vi "Gase und Konzentrationen splitten.vi"(11 "Empfangsdaten (Eingang)":string[](array[string])) -> (1 "Konzentrationen":string[](array[string]), 2 "Gase":string[](array[string]))   [LabVIEW 2020, in "Linearisierung v2.lvlib" / "Gasteiler.lvlib"]
uses:
  Gasteiler.lvlib
panel:
  # "CO2 1.729\nN2 9.983E+08\nNO2 1.729\nO2 1.642E+06\nXe 8.643E+04"
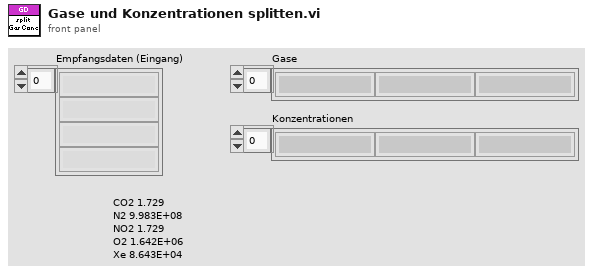
[diagram p1: front panel]
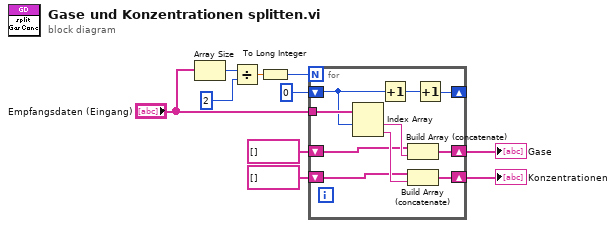
[diagram p0: block diagram]
diagram:
  n1 = Array Size(array="Empfangsdaten (Eingang)") -> (size(s)=w6:i32)
  n2 = Divide(x=w6, y=2) -> (x/y=w4:dbl)
  n3 = To Long Integer(number=w4) -> (32bit integer=w2:i32)
  n4 = for {
    N: w2 -> [_]
    tunnel: "Empfangsdaten (Eingang)" -> [w20]
    shift-right: [w17] -> w9
    shift-left: string[] [] -> [w15]
    shift-right: [w16] -> w10
    shift-left: string[] [] -> [w14]
    shift-right: [w12] -> _
    shift-left: 0 ("y") -> [w11]
    n5 = Index Array(array=w20, index #1=w11) -> (element #1=w19:string, element #2=w18:string)  [unwired: 1 in]
    n6 = Increment(x=w11) -> (x+1=w13:i32)
    n7 = Build Array (concatenate)(w15, w19) -> (w17:string[])
    n8 = Build Array (concatenate)(w14, w18) -> (w16:string[])
    n9 = Increment(x=w13) -> (x+1=w12:i32)
  }
  "Konzentrationen" <- w10
  "Gase" <- w9
